vi "Write Emergency Button.vi"(8 "error in (no error)":errorcluster, 10 "Emergency Button":refnum<vi>, 11 "User Console in":refnum<class "User Console.lvclass">) -> (0 "error out":errorcluster, 3 "User Console out":refnum<class "User Console.lvclass">)   [LabVIEW 2019]
uses:
  User Console.lvclass
  C:/Workspace/CLA/Elevator AF/Abstract User Console Actor/Abstract User Console Actor/Abstract User Console.lvclass
  C:/Program Files (x86)/National Instruments/LabVIEW 2019/vi.lib/ActorFramework/Actor/Actor.lvclass
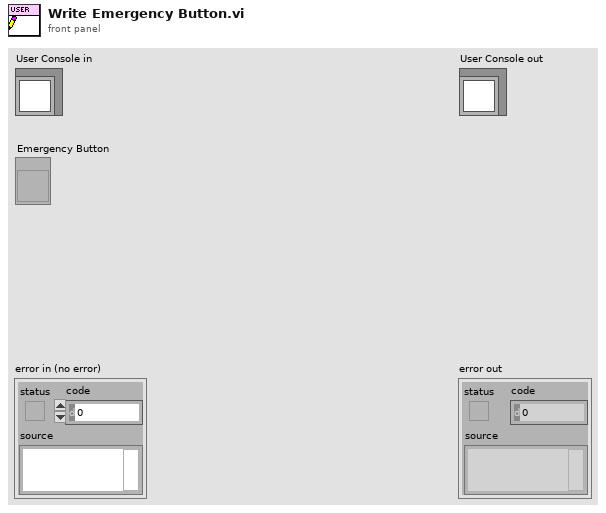
[diagram p1: front panel]
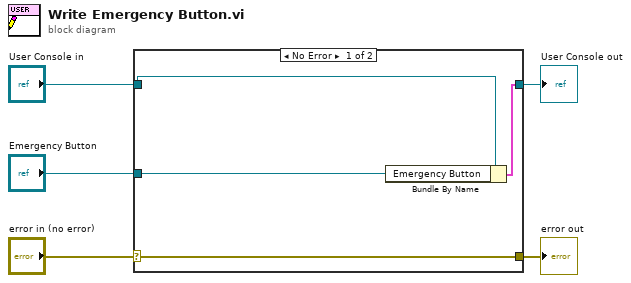
[diagram p0: block diagram]
diagram:
  n1 = case shown="No Error" "error in (no error)" {
    selector: "error in (no error)" -> [w9 w10]
    tunnel: [w9 w10] -> w4
    tunnel: [w7 w11] -> w2
    tunnel: "User Console in" -> [w8 w11]
    tunnel: "Emergency Button" -> [w6 _]
    frame No Error {
      n2 = Bundle By Name(cluster=w8, "Emergency Button"=w6) -> (w7:cluster{})
    }
    frame Error {
    }
  }
  "error out" <- w4
  "User Console out" <- w2
